vi "Find Delta Samples of Rising Edge_DBL.vi"(9 "Trigger Level":dbl=0.5 format="%#_13g", 10 "Channel 2":dbl[](array[numeric]), 11 "Channel 1":dbl[](array[numeric])) -> (3 "Sample Offset":dbl)   [LabVIEW 2026]
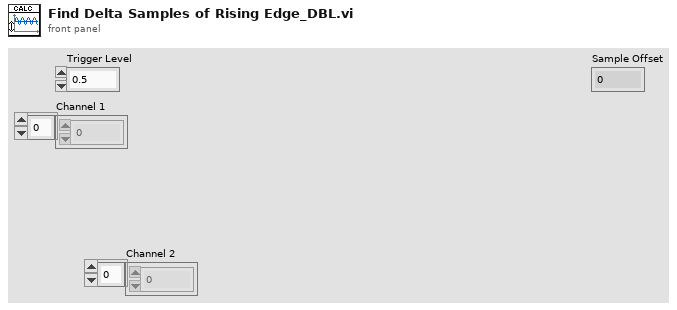
[diagram p1: front panel]
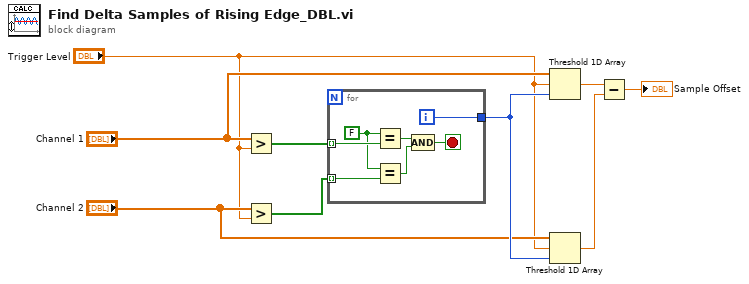
[diagram p0: block diagram]
diagram:
  n1 = Greater?(x="Channel 1", y="Trigger Level") -> (0:w6:bool[])
  n2 = Greater?(x="Channel 2", y="Trigger Level") -> (0:w5:bool[])
  n3 = for {
    tunnel: w6 -> [w16] mode=indexing
    tunnel: w5 -> [w15] mode=indexing
    tunnel: [w14] -> w4
    i -> [w14]
    stop <- w11 stop-if-true
    w10 = FALSE ("x")
    n4 = Equal?(x=w10, y=w16) -> (x = y?=w13:bool)
    n5 = Equal?(x=w10, y=w15) -> (x = y?=w12:bool)
    n6 = Compound Arithmetic op=AND(w13, w12) -> (w11:bool)
  }
  n7 = Threshold 1D Array(1:w4, 2:"Trigger Level", 3:"Channel 1") -> (0:w9:dbl)
  n8 = Threshold 1D Array(1:w4, 2:"Trigger Level", 3:"Channel 2") -> (0:w8:dbl)
  n9 = Subtract(x=w9, y=w8) -> (x-y=→"Sample Offset":dbl)
